vi "DAQmx Stop.vi"(8 "error in (no error)":errorcluster, 11 "DAQmx Container":T1) -> (0 "error out":errorcluster)   [LabVIEW 2024]
doc: "Stops the acquisition."
uses:
  support/Control/DAQmx Container.ctl
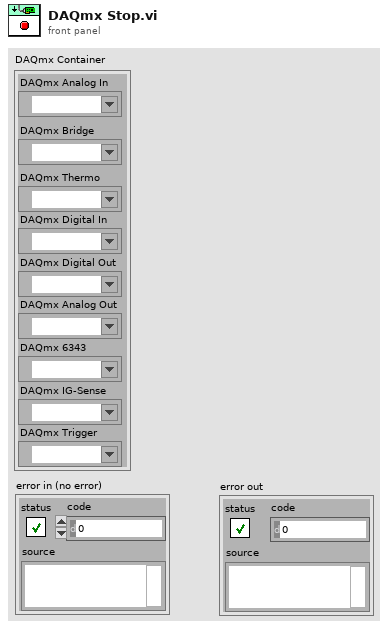
[diagram p1: front panel]
types:
  T1 = typedef "DAQmx Container.ctl" = cluster{"DAQmx Analog In":refnum<k21>, "DAQmx Digital In":refnum<k21>, "DAQmx Digital Out":refnum<k21>, "DAQmx Analog Out":refnum<k21>, "DAQmx 6343":refnum<k21>, "DAQmx IG-Sense":refnum<k21>, "DAQmx Thermo":refnum<k21>, "DAQmx Bridge":refnum<k21>, "DAQmx Trigger":refnum<k21>}
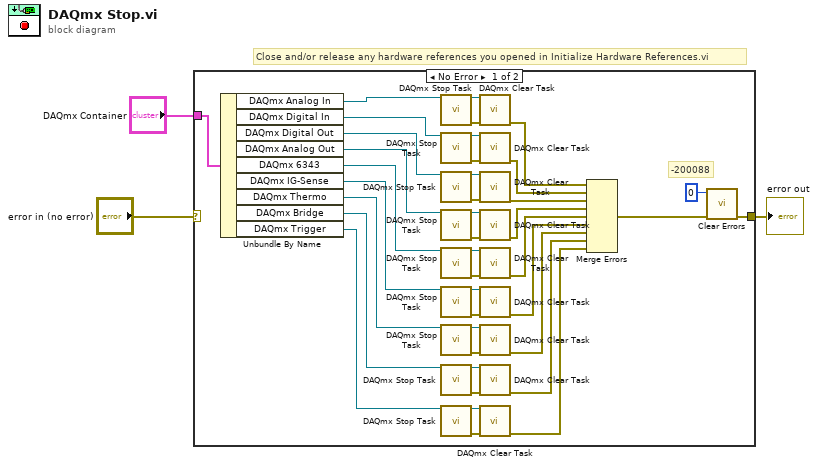
[diagram p0: block diagram]
diagram:
  # "Close and/or release any hardware references you opened in Initialize Hardware References.vi"
  n1 = case shown="No Error" "error in (no error)" {
    selector: "error in (no error)" -> [_ w44]
    tunnel: [w5 w44] -> w2
    tunnel: "DAQmx Container" -> [w42 _]
    frame No Error {
      # "-200088"
      n2 = Unbundle By Name(w42) -> ("DAQmx Analog In"=w41:refnum<k21>, "DAQmx Digital In"=w36:refnum<k21>, "DAQmx Digital Out"=w34:refnum<k21>, "DAQmx Analog Out"=w23:refnum<k21>, "DAQmx 6343"=w22:refnum<k21>, "DAQmx IG-Sense"=w21:refnum<k21>, "DAQmx Thermo"=w18:refnum<k21>, "DAQmx Bridge"=w11:refnum<k21>, "DAQmx Trigger"=w6:refnum<k21>)
      n3 = call <vilib>:"DAQmx Stop Task.vi"("task/channels in"=w41) -> ("task out"=w40:refnum<k21>, "error out"=w39:errorcluster)  [unwired: 13 in]
      n4 = call <vilib>:"DAQmx Stop Task.vi"("task/channels in"=w36) -> ("task out"=w37:refnum<k21>, "error out"=w38:errorcluster)  [unwired: 13 in]
      n5 = call <vilib>:"DAQmx Stop Task.vi"("task/channels in"=w34) -> ("task out"=w30:refnum<k21>, "error out"=w35:errorcluster)  [unwired: 13 in]
      n6 = call <vilib>:"DAQmx Stop Task.vi"("task/channels in"=w23) -> ("task out"=w29:refnum<k21>, "error out"=w28:errorcluster)  [unwired: 13 in]
      n7 = call <vilib>:"DAQmx Stop Task.vi"("task/channels in"=w22) -> ("task out"=w26:refnum<k21>, "error out"=w27:errorcluster)  [unwired: 13 in]
      n8 = call <vilib>:"DAQmx Stop Task.vi"("task/channels in"=w21) -> ("task out"=w24:refnum<k21>, "error out"=w25:errorcluster)  [unwired: 13 in]
      n9 = call <vilib>:"DAQmx Stop Task.vi"("task/channels in"=w18) -> ("task out"=w19:refnum<k21>, "error out"=w20:errorcluster)  [unwired: 13 in]
      n10 = call <vilib>:"DAQmx Stop Task.vi"("task/channels in"=w11) -> ("task out"=w12:refnum<k21>, "error out"=w13:errorcluster)  [unwired: 13 in]
      n11 = call <vilib>:"DAQmx Stop Task.vi"("task/channels in"=w6) -> ("task out"=w8:refnum<k21>, "error out"=w9:errorcluster)  [unwired: 13 in]
      n12 = call <vilib>:"DAQmx Clear Task.vi"("task in"=w40, "error in"=w39) -> ("error out"=w33:errorcluster)  [unwired: 13 in]
      n13 = call <vilib>:"DAQmx Clear Task.vi"("task in"=w37, "error in"=w38) -> ("error out"=w32:errorcluster)  [unwired: 13 in]
      n14 = call <vilib>:"DAQmx Clear Task.vi"("task in"=w30, "error in"=w35) -> ("error out"=w31:errorcluster)  [unwired: 13 in]
      n15 = call <vilib>:"DAQmx Clear Task.vi"("task in"=w29, "error in"=w28) -> ("error out"=w17:errorcluster)  [unwired: 13 in]
      n16 = call <vilib>:"DAQmx Clear Task.vi"("task in"=w26, "error in"=w27) -> ("error out"=w16:errorcluster)  [unwired: 13 in]
      n17 = call <vilib>:"DAQmx Clear Task.vi"("task in"=w24, "error in"=w25) -> ("error out"=w15:errorcluster)  [unwired: 13 in]
      n18 = call <vilib>:"DAQmx Clear Task.vi"("task in"=w19, "error in"=w20) -> ("error out"=w14:errorcluster)  [unwired: 13 in]
      n19 = call <vilib>:"DAQmx Clear Task.vi"("task in"=w12, "error in"=w13) -> ("error out"=w10:errorcluster)  [unwired: 13 in]
      n20 = call <vilib>:"DAQmx Clear Task.vi"("task in"=w8, "error in"=w9) -> ("error out"=w7:errorcluster)  [unwired: 13 in]
      n21 = Merge Errors(w33, w32, w31, w17, w16, w15, w14, w10, w7) -> (w43:errorcluster)
      n22 = call <vilib>:"Clear Errors.vi"("error in (no error)"=w43, "specific error code to clear (0: all)"=0) -> ("error out"=w5:errorcluster)  [unwired: 4 in, 1 out]
    }
    frame Error {
    }
  }
  "error out" <- w2
